vi "Test Initializing.vi"() -> ()   [LabVIEW 2015, in "Numeric Limit Compare Tests.lvlib"]
uses:
  Numeric Limit Compare Tests.lvlib
  classes/Sequence/Config/Sequence Config.lvclass
  Config/Numeric Limit Compare Config.lvclass
  Config/Comparison Types.ctl
  <vilib>/NI/Tag Bus/tag/Data Type.ctl
  <vilib>/NI/Tag Bus Module Framework/channel/channel classification.ctl
  Config/Numeric Limit Compare Config.lvclass/Numeric Limit Compare Config.ctl
  Config/Write Comparison Type.vi
  Config/Write Lower Limit.vi
  Config/Write Negate Result.vi
  Config/Write Result Channel.vi
  Config/Write channel.vi
  Config/Write Upper Limit_Limit.vi
  classes/Sequence/Execution/Sequence.lvclass
  <vilib>/NI/Tag Bus Module Framework/channel/TBM channel.lvclass
  <vilib>/NI/Tag Bus/tag/tag descriptor.lvclass
panel:
  out "error out":errorcluster
  out "Pass":bool
  out "Name":string
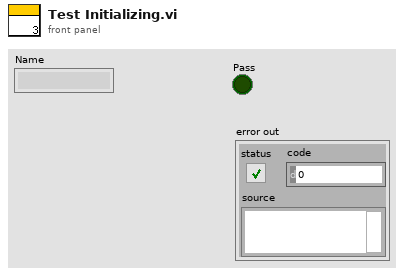
[diagram p1: front panel]
types:
  T1 = typedef "TBM channel.lvclass/channel classification.ctl" = enum16{"input data", "output data", "processing parameter", "processing result"}
  T2 = typedef "tag bus.lvlib/tag descriptor.lvclass/Data Type.ctl" = enum16{"Double", "Single", "I64", "I32", "I16", "I8", "U64", "U32", "U16", "U8", "Boolean", "String", "Array of Double", "Array of Single", "Array of I64", "Array of I32", "Array of I16", "Array of I8", "Array of U64", "Array of U32", "Array of U16", "Array of U8", "Array of Boolean", "Array of String"}
  T3 = typedef "Comparison Types.ctl" = enum16{"GELE (>=<=)", "GTLE(><=)", "GTLT(><)", "GELT(>=<)", "EQ(==)", "NE (!=)", "GT(>)", "LT(<)", "GE(>=)", "LE(<=)"}
  T4 = typedef "TBM channel.lvclass/data tables.ctl" = cluster{"input data":T5, "processing parameter":T5, "processing result":T5, "output data":T5}
  T5 = typedef "tag bus.lvlib/dictionary table pair.ctl" = cluster{"data dictionary":refnum<class "data dictionary.lvclass">, "data table":T6}
  T6 = typedef "tag bus.lvlib/data table.lvlib/data table.ctl" = cluster{"Double":dbl[], "Single":sgl[], "I64":i64[], "I32":i32[], "I16":i16[], "I8":i8[], "U64":u64[], "U32":u32[], "U16":u16[], "U8":u8[], "Boolean":bool[], "String":string[], "Array of Double":cluster{"DBL Array":dbl[]}[], "Array of Single":cluster{"SGL Array":sgl[]}[], "Array of I64":cluster{"I64 Array":i64[]}[], "Array of I32":cluster{"I32 Array":i32[]}[], "Array of I16":cluster{"I16 Array":i16[]}[], "Array of I8":cluster{"I8 Array":i8[]}[], "Array of U64":cluster{"U64 Array":u64[]}[], "Array of U32":cluster{"U32 Array":u32[]}[], "Array of U16":cluster{"U16 Array":u16[]}[], "Array of U8":cluster{"U8 Array":u8[]}[], "Array of Boolean":cluster{"Boolean Array":bool[]}[], "Array of String":cluster{"String Array":string[]}[]}
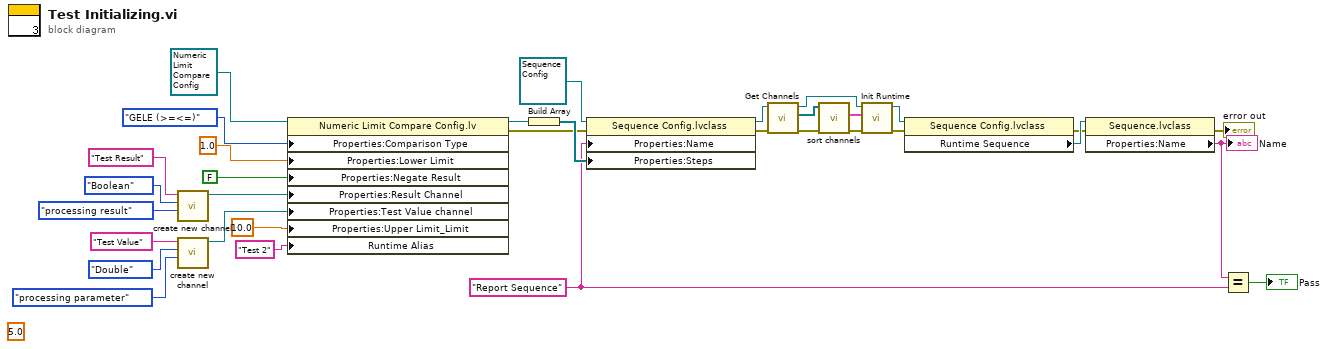
[diagram p0: block diagram]
diagram:
  (unwired) 5.0 ("Upper Limit_Limit")
  w3 = "Report Sequence" ("Name")
  n1 = call <vilib>:"create new channel.vi"("channel classification"=channel_classification."processing result", "data type"=Data_Type."Boolean", "channel name"="Test Result") -> ("channel"=w13:refnum<class "TBM channel.lvclass">)  [unwired: 8 in]
  n2 = call <vilib>:"create new channel.vi"("channel classification"=channel_classification."processing parameter", "data type"=Data_Type."Double", "channel name"="Test Value") -> ("channel"=w17:refnum<class "TBM channel.lvclass">)  [unwired: 8 in]
  n3 = property class="Numeric Limit Compare Config.lv"(reference=refnum<class "Numeric Limit Compare Config.lvclass"> refnum ("Numeric Limit Compare Config.lvclass"), "Properties:Comparison Type"=Comparison_Types."GELE (>=<=)" ("Comparison Type"), "Properties:Lower Limit"=1.0 ("Lower Limit"), "Properties:Negate Result"=FALSE ("Negate Result"), "Properties:Result Channel"=w13, "Properties:Test Value channel"=w17, "Properties:Upper Limit_Limit"=10.0 ("Upper Limit_Limit"), "Runtime Alias"="Test 2") -> (reference out=w18:refnum<class "Numeric Limit Compare Config.lvclass">, error out=w8:errorcluster)  [unwired: 1 in]
  n4 = Build Array(w18) -> (w25:refnum<class "Numeric Limit Compare Config.lvclass">[])
  n5 = property class="Sequence Config.lvclass"(reference=refnum<class "Sequence Config.lvclass"> refnum ("Sequence Config.lvclass"), error in=w8, "Properties:Name"=w3, "Properties:Steps"=w25) -> (reference out=w9:refnum<class "Sequence Config.lvclass">, error out=w6:errorcluster)
  n6 = call "Get Channels.vi"("error in (no error)"=w6, "Sequence Config in"=w9) -> ("error out"=w30:errorcluster, "Channels"=w32:refnum<class "TBM channel.lvclass">[], "Sequence Config out"=w33:refnum<class "Sequence Config.lvclass">)  [unwired: 7 in]
  n7 = call <vilib>:"sort channels.vi"("error in"=w30, "channels in"=w32) -> ("error out"=w29:errorcluster, "data allocations"=w31:T4)  [unwired: 7 in, 1 out]
  n8 = call-dynamic "Init Runtime.vi"("error in (no error)"=w29, "data allocations"=w31, "Sequence Config in"=w33) -> ("error out"=w7:errorcluster, "Sequence Config out"=w28:refnum<class "Sequence Config.lvclass">)  [unwired: 7 in]
  n9 = property class="Sequence Config.lvclass"(reference=w28, error in=w7) -> (error out=w5:errorcluster, "Runtime Sequence"=w27:refnum<class "Sequence.lvclass">)  [unwired: 1 out]
  n10 = property class="Sequence.lvclass"(reference=w27, error in=w5) -> (error out=→"error out":errorcluster, "Properties:Name"=w4:string)  [unwired: 1 out]
  "Name" <- w4
  n11 = Equal?(x=w4, y=w3) -> (x = y?=→"Pass":bool)
